vi "Get Standoff Position.vi"(7 "Direction":enum16{"- infinity", "+ infinity"}(ring)=enum."+ infinity", 8 "error in (no error)":errorcluster, 9 "Timeout (sec)":dbl=100.0, 10 "Index":i32, 11 "Visa Array in":refnum<visa-resource-name>[](array[refnum])) -> (0 "error out":errorcluster, 1 "Time out":bool, 2 "Standoff":dbl, 3 "Visa Array out":refnum<visa-resource-name>[](array[refnum]))   [LabVIEW 2010, in "SignalWriterMH110203USBStepperMotor.lvclass"]
uses:
  SignalWriterMH110203USBStepperMotor.lvclass
  class_data.vi
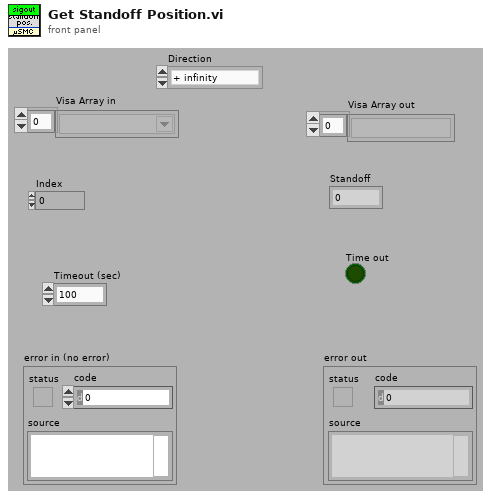
[diagram p1: front panel]
types:
  T1 = typedef "SignalWriterMH110203USBStepperMotor.lvclass/Get State Control (uSMC).ctl" = cluster{"Current Posistion":dbl, "CW/CCW":bool, "Speed":u16, "Temperature":dbl, "Power":u16, "Limit Switch 1":bool, "Limit Switch 2":bool, "After Reset":bool, "Step":u8, "Backlash":bool, "RT Error":bool, "RT State":bool, "Sync In":bool, "Sync Out":bool, "Ext Disconnect":bool, "Usb Powered":bool, "Voltage":dbl, "Working":bool, "SM Position in Encoder Units":i32, "Encoder Current Position":i32}
  T2 = typedef "SignalWriterMH110203USBStepperMotor.lvclass/GoTo Control (uSMC).ctl" = cluster{"Step motor ID":string, "SMname":string, "Backlash":u16, "wait for input sygnal to start":bool, "use slow start/stop":bool, "units name":string, "Maximum speed":dbl, "speed":dbl, "step":u8, "point 1 ticks":i32, "point 2 ticks":i32, "point 1 units":dbl, "point 2 units":dbl, "Limit Switch standoff":dbl, "Zero Value":dbl, "Destination Position":dbl, "force backlash":bool, "power off when stop":bool, "POff delay":dbl, "positioner name":string, "R, Ohm":dbl, "I, mA":dbl, "Positioner's Type":u16, "Reset Direction":bool, "Manufacturer":string, "Model":string, "Scheme":string, "FirmwareVer":string}
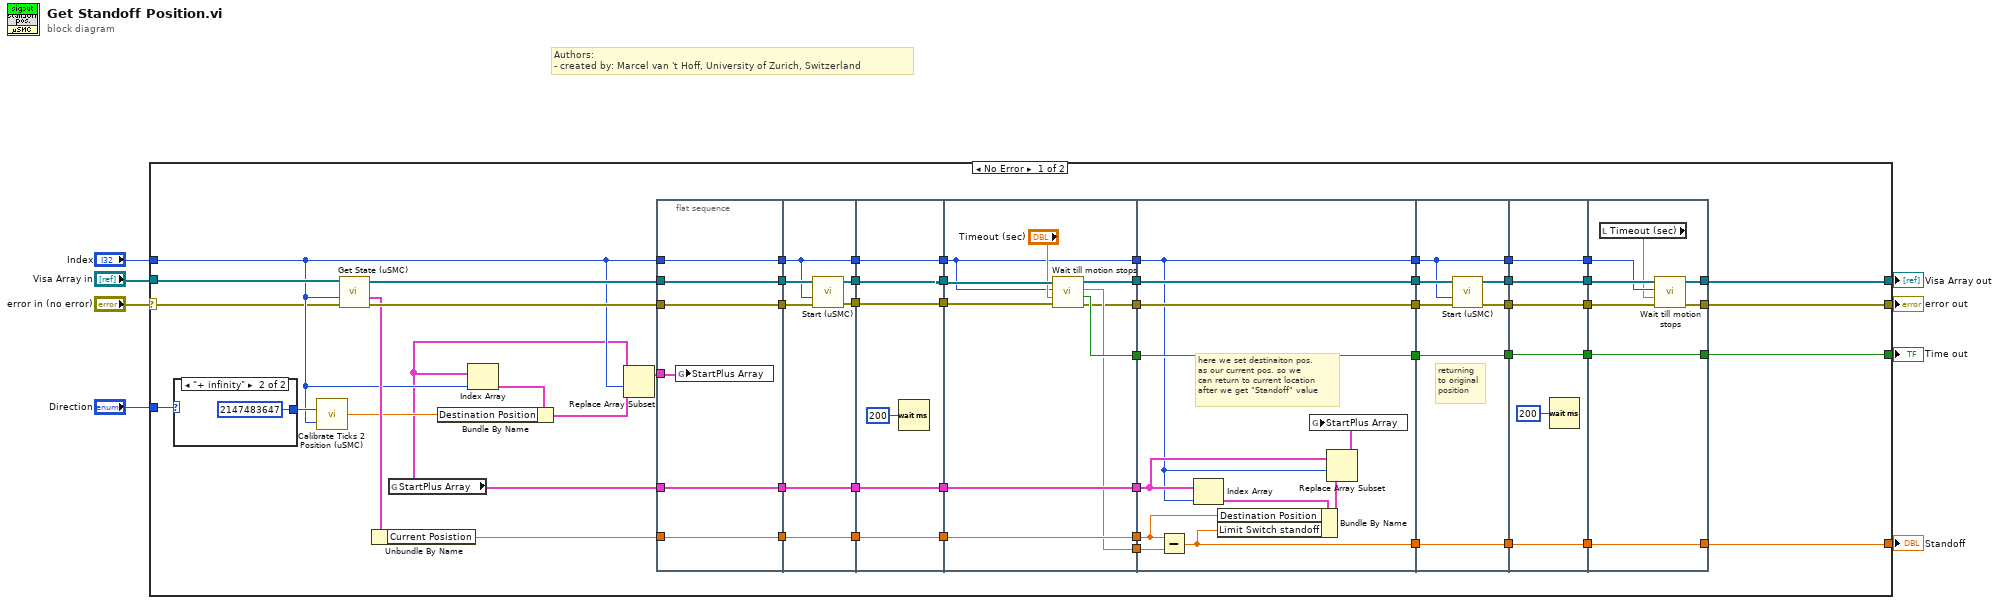
[diagram p0: block diagram]
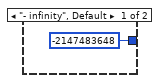
[diagram p2: hidden frame]
diagram:
  # "Authors: \n- created by: Marcel van 't Hoff, University of Zurich, Switzerland"
  n1 = case shown="No Error" "error in (no error)" {
    selector: "error in (no error)" -> [w20 w128]
    tunnel: "Visa Array in" -> [w35 w127]
    tunnel: "Direction" -> [w31 _]
    tunnel: "Index" -> [w25 _]
    tunnel: [w19 w127] -> w5
    tunnel: [w24 w128] -> w4
    tunnel: [w23 _] -> w3
    tunnel: [w22 _] -> w2
    frame No Error {
      n2 = case shown="\"+ infinity\"" w31 {
        tunnel: [-2147483648 ("ticks") 2147483647 ("ticks")] -> w30
        frame "- infinity", Default {
        }
        frame "+ infinity" {
        }
      }
      n3 = call "Calibrate Ticks 2 Position (uSMC).vi"("array index"=w25, "ticks"=w30) -> ("value"=w29:dbl)
      n4 = call "Get State (uSMC).vi"("error in (no error)"=w20, "SM number"=w25, "Visa array in"=w35) -> ("error out"=w33:errorcluster, "State cluster"=w32:T1, "Visa array out"=w34:refnum<visa-resource-name>[])  [unwired: 6 in]
      n5 = Unbundle By Name(w32) -> ("Current Posistion"=w26:dbl)
      n6 = global read "class_data.vi" "StartPlus Array"() -> (w21:T2[])
      n7 = Index Array(array=w21, index=w25) -> (element=w27:T2)
      n8 = Bundle By Name(cluster=w27, "Destination Position"=w29) -> (w28:T2)
      n9 = Replace Array Subset(array=w21, new element=w28, index=w25) -> (w36:T2[])
      n10 = flat-sequence {
        tunnel: w25 -> [w69]
        tunnel: w33 -> [w70]
        tunnel: w34 -> [w71]
        tunnel: [w71] -> w63
        tunnel: [w70] -> w62
        tunnel: [w69] -> w61
        tunnel: w36 -> [w68]
        tunnel: [w67] -> w60
        tunnel: w21 -> [w67]
        tunnel: [w66] -> w59
        tunnel: w26 -> [w66]
        tunnel: w63 -> [w78]
        tunnel: w62 -> [w76]
        tunnel: w61 -> [w74]
        tunnel: [w77] -> w58
        tunnel: [w75] -> w57
        tunnel: [w74] -> w56
        tunnel: [w73] -> w55
        tunnel: w60 -> [w73]
        tunnel: [w72] -> w54
        tunnel: w59 -> [w72]
        tunnel: w58 -> [w84]
        tunnel: w57 -> [w83]
        tunnel: w56 -> [w82]
        tunnel: [w84] -> w53
        tunnel: [w83] -> w52
        tunnel: [w82] -> w51
        tunnel: [w81] -> w50
        tunnel: w55 -> [w81]
        tunnel: [w80] -> w49
        tunnel: w54 -> [w80]
        tunnel: w53 -> [w92]
        tunnel: w52 -> [w90]
        tunnel: w51 -> [w88]
        tunnel: [w91] -> w48
        tunnel: [w85] -> w47
        tunnel: [w94] -> w46
        tunnel: w50 -> [w94]
        tunnel: [w93] -> w45
        tunnel: w49 -> [w93]
        tunnel: [w86] -> w44
        tunnel: [w88] -> w43
        tunnel: [w87] -> w42
        tunnel: w48 -> [w105]
        tunnel: w47 -> [w104]
        tunnel: w46 -> [w96]
        tunnel: w45 -> [w98]
        tunnel: w44 -> [w103]
        tunnel: [w105] -> w41
        tunnel: [w104] -> w40
        tunnel: [w95] -> w39
        tunnel: w43 -> [w95]
        tunnel: [w97] -> w38
        tunnel: [w102] -> w37
        tunnel: w42 -> [w102]
        tunnel: w41 -> [w112]
        tunnel: w40 -> [w111]
        tunnel: w39 -> [w106]
        tunnel: w38 -> [w108]
        tunnel: w37 -> [w107]
        tunnel: [w110] -> w18
        tunnel: [w109] -> w17
        tunnel: [w108] -> w16
        tunnel: [w107] -> w15
        tunnel: [w106] -> w10
        tunnel: w18 -> [w118]
        tunnel: w17 -> [w117]
        tunnel: w16 -> [w116]
        tunnel: w15 -> [w115]
        tunnel: [w118] -> w14
        tunnel: [w117] -> w13
        tunnel: [w116] -> w12
        tunnel: [w115] -> w11
        tunnel: w10 -> [w113]
        tunnel: [w113] -> w9
        tunnel: [w125] -> w22
        tunnel: [w126] -> w23
        tunnel: [w121] -> w24
        tunnel: [w122] -> w19
        tunnel: w14 -> [w123]
        tunnel: w13 -> [w124]
        tunnel: w12 -> [w126]
        tunnel: w11 -> [w125]
        tunnel: w9 -> [w120]
        frame #0 {
          n11 = global write "class_data.vi" "StartPlus Array"(w68) -> ()
        }
        frame #1 {
          n12 = call "Start (uSMC).vi"("error in"=w76, "Index"=w74, "Visa Array In"=w78) -> ("error out"=w75:errorcluster, "Visa Array Out"=w77:refnum<visa-resource-name>[])  [unwired: 7 in]
        }
        frame #2 {
          n13 = Wait (ms)(milliseconds to wait=u32 200) -> ()  [unwired: 1 out]
        }
        frame #3 {
          n14 = call "Wait till motion stops.vi"("error in"=w90, "Timeout (sec)"="Timeout (sec)", "Index"=w88, "Visa Array Out"=w92) -> ("error out"=w85:errorcluster, "Time out?"=w87:bool, "Current Posistion"=w86:dbl, "Visa array out"=w91:refnum<visa-resource-name>[])  [unwired: 4 in]
        }
        frame #4 {
          # "here we set destinaiton pos.\nas our current pos. so we\ncan return to current location\nafter we get \"Standoff\" value"
          n15 = Subtract(x=w98, y=w103) -> (x-y=w97:dbl)
          n16 = Index Array(array=w96, index=w95) -> (element=w100:T2)
          n17 = Bundle By Name(cluster=w100, "Destination Position"=w98, "Limit Switch standoff"=w97) -> (w101:T2)
          n18 = Replace Array Subset(array=w96, new element=w101, index=w95) -> (w99:T2[])
          n19 = global write "class_data.vi" "StartPlus Array"(w99) -> ()
        }
        frame #5 {
          # "returning\nto original\nposition"
          n20 = call "Start (uSMC).vi"("error in"=w111, "Index"=w106, "Visa Array In"=w112) -> ("error out"=w109:errorcluster, "Visa Array Out"=w110:refnum<visa-resource-name>[])  [unwired: 7 in]
        }
        frame #6 {
          n21 = Wait (ms)(milliseconds to wait=u32 200) -> ()  [unwired: 1 out]
        }
        frame #7 {
          n22 = local read "Timeout (sec)"() -> (w119:dbl)
          n23 = call "Wait till motion stops.vi"("error in"=w124, "Timeout (sec)"=w119, "Index"=w120, "Visa Array Out"=w123) -> ("error out"=w121:errorcluster, "Visa array out"=w122:refnum<visa-resource-name>[])  [unwired: 4 in, 2 out]
        }
      }
    }
    frame Error {
    }
  }
  "Visa Array out" <- w5
  "error out" <- w4
  "Standoff" <- w3
  "Time out" <- w2
